vi "Cryomagnetics Set Sweep Mode.vi"(8 "error in (no error)":errorcluster, 10 "sweep mode":T1, 11 "VISA Resource Name":refnum<visa-resource-name>) -> (0 "error out":errorcluster, 3 "VISA Resource Name Out":refnum<visa-resource-name>)   [LabVIEW 2015]
uses:
  Sweep mode.ctl
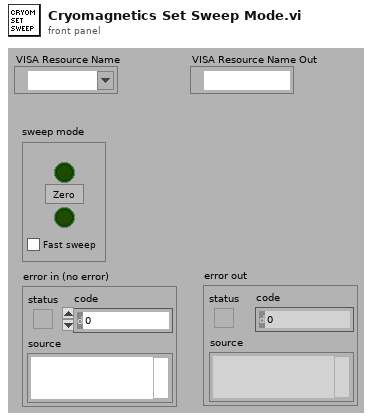
[diagram p1: front panel]
types:
  T1 = typedef "Sweep mode.ctl" = cluster{"zero":bool, "sweep up":bool, "sweep down":bool, "fast sweep":bool}
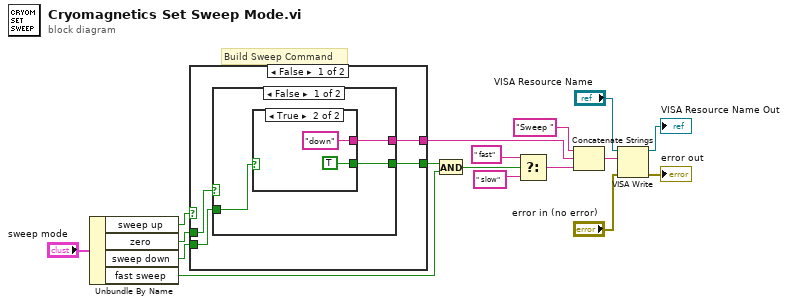
[diagram p0: block diagram]
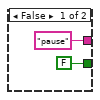
[diagram p2: hidden frame]
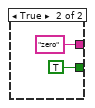
[diagram p3: hidden frame]
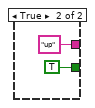
[diagram p4: hidden frame]
diagram:
  # "Build Sweep Command"
  n1 = Unbundle By Name("sweep mode") -> ("sweep up"=w17:bool, "zero"=w16:bool, "sweep down"=w15:bool, "fast sweep"=w13:bool)
  n2 = case shown="False" w17 {
    tunnel: [w20 "up"] -> w8
    tunnel: w16 -> [w21 _]
    tunnel: w15 -> [w19 _]
    tunnel: [w18 TRUE] -> w14
    frame False {
      n3 = case shown="False" w21 {
        tunnel: [w24 "zero"] -> w20
        tunnel: w19 -> [w22 _]
        tunnel: [w23 TRUE] -> w18
        frame False {
          n4 = case shown="True" w22 {
            tunnel: ["pause" "down"] -> w24
            tunnel: [FALSE TRUE] -> w23
            frame False {
            }
            frame True {
            }
          }
        }
        frame True {
        }
      }
    }
    frame True {
    }
  }
  n5 = And(x=w14, y=w13) -> (x .and. y?=w12:bool)
  n6 = Select(t=" fast", s=w12, f=" slow") -> (s? t:f=w7:string)
  n7 = Concatenate Strings("Sweep ", w8, w7) -> (w1:string)
  n8 = VISA Write(VISA resource name="VISA Resource Name", write buffer=w1, error in (no error)="error in (no error)") -> (VISA resource name out=→"VISA Resource Name Out":refnum<visa-resource-name>, error out=→"error out":errorcluster)  [unwired: 1 out]
